vi "Bool_Delay OnOFF.vi"(7 "Delay Time(S)":dbl=2.0, 10 "Delay On(t) Off(f)":bool=TRUE, 11 "Input":bool) -> (3 "Output":bool, 5 "Time Remaining":dbl)   [LabVIEW 2020]
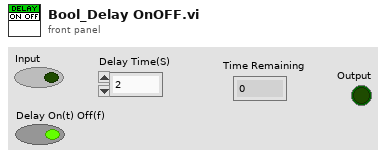
[diagram p1: front panel]
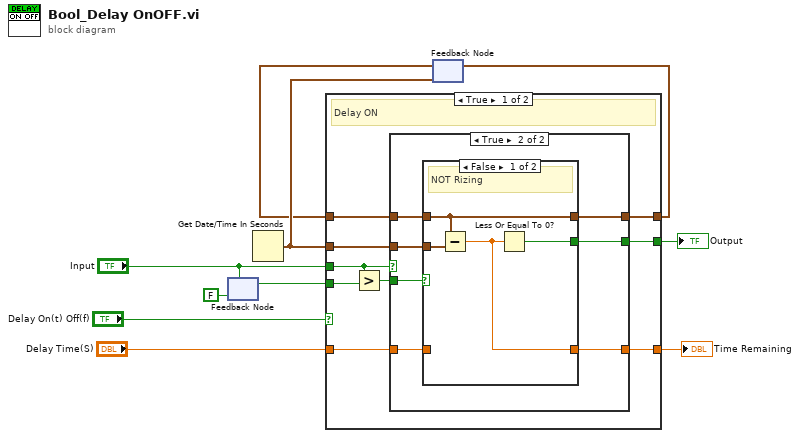
[diagram p0: block diagram]
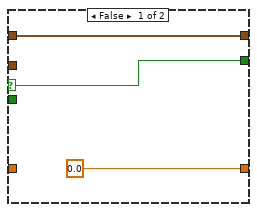
[diagram p2: hidden frame]
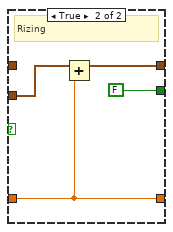
[diagram p3: hidden frame]
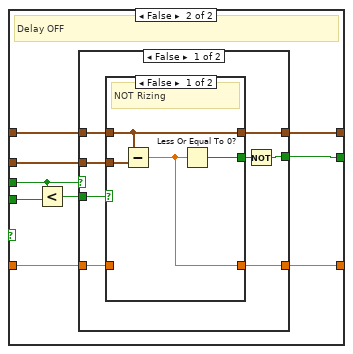
[diagram p4: hidden frame]
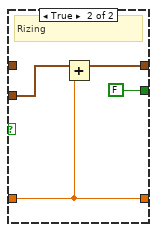
[diagram p5: hidden frame]
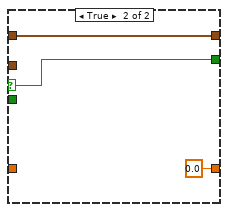
[diagram p6: hidden frame]
diagram:
  n1 = feedback #1(FALSE ("Input")) -> (w9:bool)
  n2 = feedback-in #1("Input") -> ()
  n3 = Get Date/Time In Seconds() -> (seconds since 1Jan1904=w6:timestamp)
  n4 = feedback #2(w6) -> (w5:timestamp)
  n5 = case shown="True" "Delay On(t) Off(f)" {
    tunnel: w9 -> [w19 w46]
    tunnel: "Input" -> [w11 w40]
    tunnel: w6 -> [w15 w43]
    tunnel: [w16 w44] -> w7
    tunnel: w5 -> [w17 w39]
    tunnel: [w14 w38] -> w4
    tunnel: "Delay Time(S)" -> [w13 w42]
    tunnel: [w12 w41] -> w2
    frame True {
      # "Delay ON"
      n6 = Greater?(x=w11, y=w19) -> (0:w18:bool)
      n7 = case shown="True" w11 {
        selector: w11 -> [w22 _]
        tunnel: w18 -> [_ w29]
        tunnel: w17 -> [w20 w28]
        tunnel: [w20 w27] -> w16
        tunnel: w15 -> [_ w26]
        tunnel: [w22 w25] -> w14
        tunnel: w13 -> [_ w24]
        tunnel: [0.0 ("Delay Time(S)") w23] -> w12
        frame False {
        }
        frame True {
          n8 = case shown="False" w29 {
            tunnel: w28 -> [w32 _]
            tunnel: [w32 w35] -> w27
            tunnel: w26 -> [w33 w37]
            tunnel: [w31 FALSE] -> w25
            tunnel: w24 -> [_ w34]
            tunnel: [w30 w34] -> w23
            frame False {
              # "NOT Rizing"
              n9 = Subtract(x=w32, y=w33) -> (x-y=w30:dbl)
              n10 = Less Or Equal To 0?(x=w30) -> (x <= 0?=w31:bool)
            }
            frame True {
              # "Rizing"
              n11 = Add(x=w37, y=w34) -> (x+y=w35:timestamp)
            }
          }
        }
      }
    }
    frame False {
      # "Delay OFF"
      n12 = Less?(x=w40, y=w46) -> (x < y?=w45:bool)
      n13 = case shown="False" w40 {
        selector: w40 -> [_ w63]
        tunnel: w45 -> [w54 _]
        tunnel: [w52 w65] -> w44
        tunnel: w43 -> [w51 _]
        tunnel: w42 -> [w50 _]
        tunnel: [w49 0.0 ("Delay Time(S)")] -> w41
        tunnel: w39 -> [w53 w65]
        tunnel: [w47 w63] -> w38
        frame False {
          n14 = case shown="False" w54 {
            tunnel: w53 -> [w57 _]
            tunnel: [w57 w60] -> w52
            tunnel: w51 -> [w58 w62]
            tunnel: [w56 FALSE] -> w48
            tunnel: w50 -> [_ w59]
            tunnel: [w55 w59] -> w49
            frame False {
              # "NOT Rizing"
              n15 = Subtract(x=w57, y=w58) -> (x-y=w55:dbl)
              n16 = Less Or Equal To 0?(x=w55) -> (x <= 0?=w56:bool)
            }
            frame True {
              # "Rizing"
              n17 = Add(x=w62, y=w59) -> (x+y=w60:timestamp)
            }
          }
          n18 = Not(x=w48) -> (.not. x?=w47:bool)
        }
        frame True {
        }
      }
    }
  }
  "Output" <- w4
  "Time Remaining" <- w2
  n19 = feedback-in #2(w7) -> ()
